vi "TIFF Get Write Proc.vi"(8 "error in (no error)":errorcluster, 11 "para0":cluster{}) -> (0 "error out":errorcluster, 2 "function return":u32, 3 "para0 out":cluster{})   [LabVIEW 2018]
doc: "LIBTIFF_DLL_IMPEXP TIFFReadWriteProc TIFFGetWriteProc(TIFF*);"
uses:
  libtiff3.dll
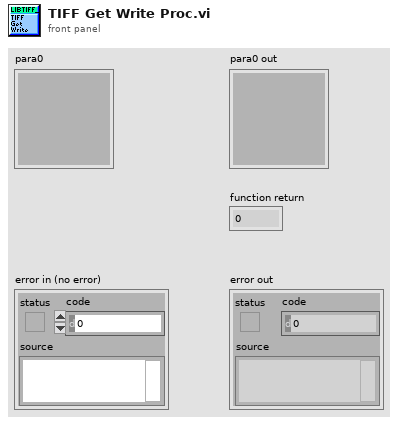
[diagram p1: front panel]
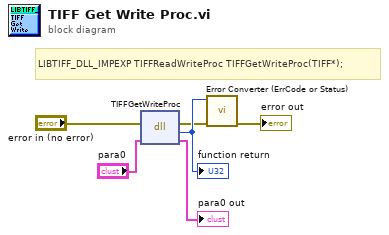
[diagram p0: block diagram]
diagram:
  # "LIBTIFF_DLL_IMPEXP\tTIFFReadWriteProc TIFFGetWriteProc(TIFF*);"
  n1 = dll-call lib="C:/Users/johan/Downloads/LabVIEW software/LabVIEW software/IX-81 Software/lib/tiff/LibTiffLabview/libtiff3.*" fn="TIFFGetWriteProc"(error in="error in (no error)", "para0"="para0") -> (error out=w2:errorcluster, w6:u32, "para0"=→"para0 out":cluster{})  [unwired: 2 in, 1 out]
  "function return" <- w6
  n2 = call "Error Converter (ErrCode or Status).vi"("error in (no error)"=w2, "error code"=w6) -> ("error out"=→"error out":errorcluster)  [unwired: 9 in]
